vi "Encode JSON Recursive.vi"(4 "error in (no error)":errorcluster, 6 "String In":string, 7 "JSON Tree":variant) -> (0 "error out":errorcluster, 2 "String Out":string)   [LabVIEW 2011, in "i3-json.lvlib"]
uses:
  i3-json.lvlib
  JSON Types/JSON Type.ctl
  Generation Error.ctl
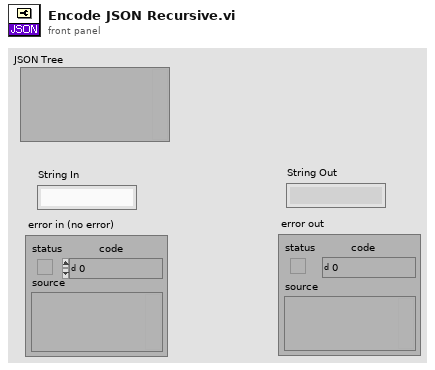
[diagram p1: front panel]
types:
  T1 = typedef "i3-json.lvlib/JSON Type.ctl" = enum8{"JSON Compatible", "JSON Array", "JSON Object", "JSON Null", "Double", "String", "Boolean", "Unknown", "Data JSON string"}
  T2 = typedef "i3-json.lvlib/Generation Error.ctl" = string
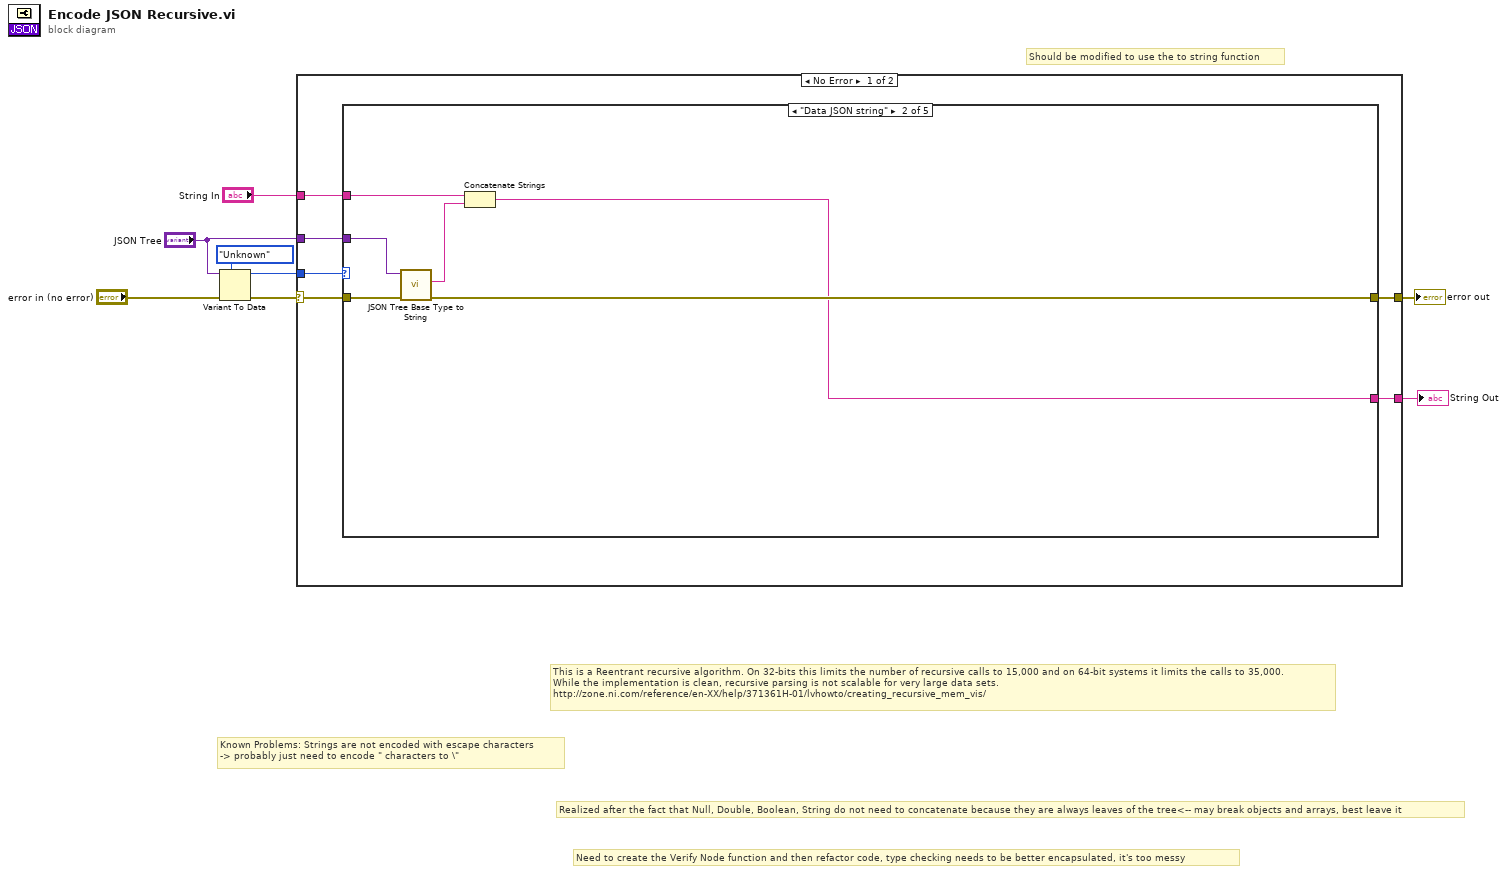
[diagram p0: block diagram]
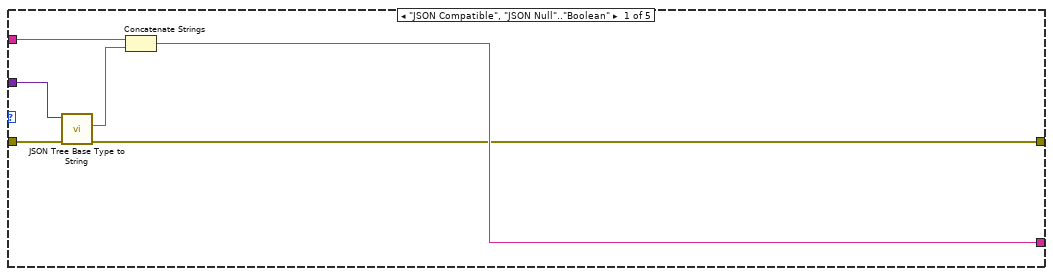
[diagram p2: hidden frame]
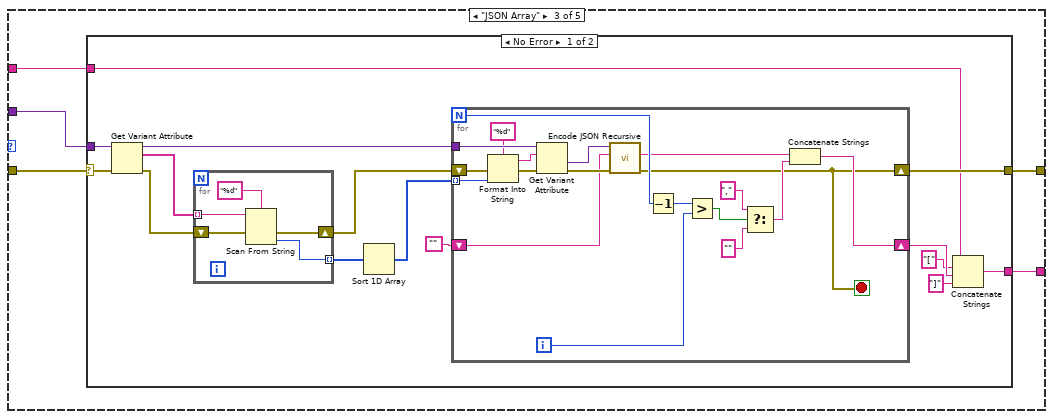
[diagram p3: hidden frame]
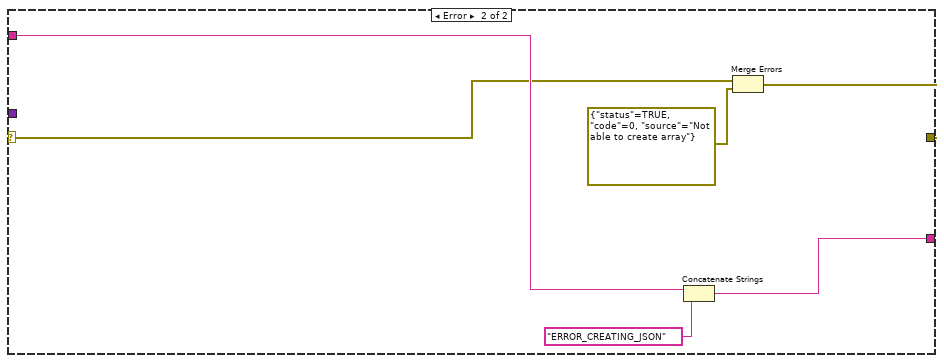
[diagram p4: hidden frame]
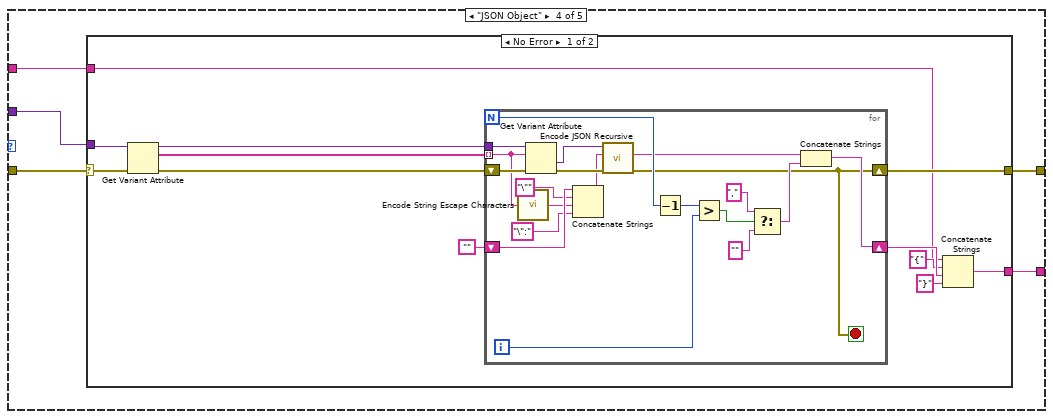
[diagram p5: hidden frame]
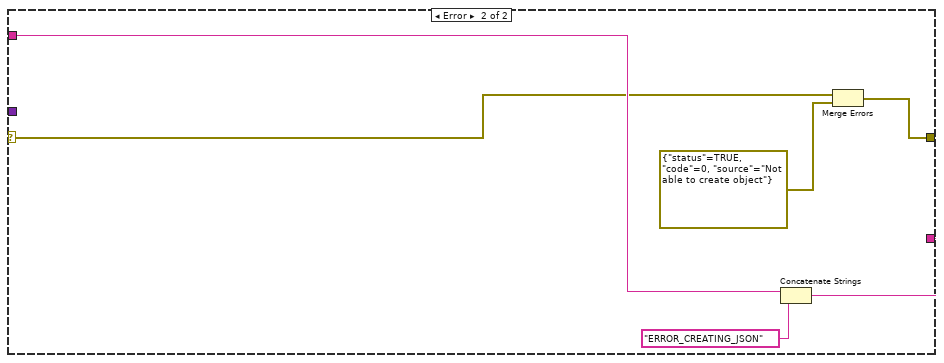
[diagram p6: hidden frame]
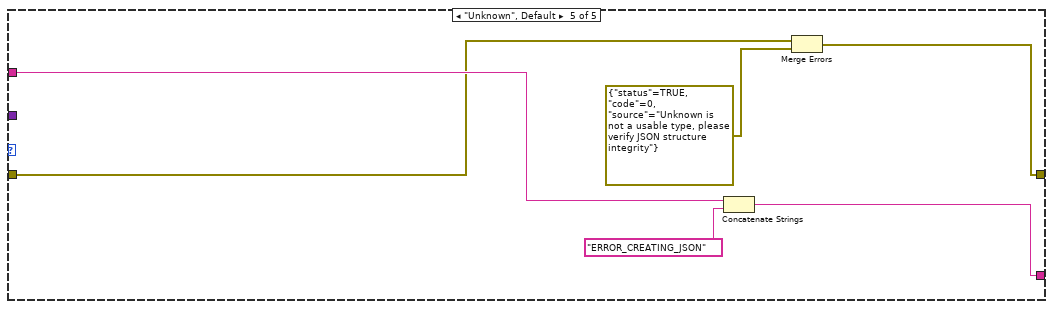
[diagram p7: hidden frame]
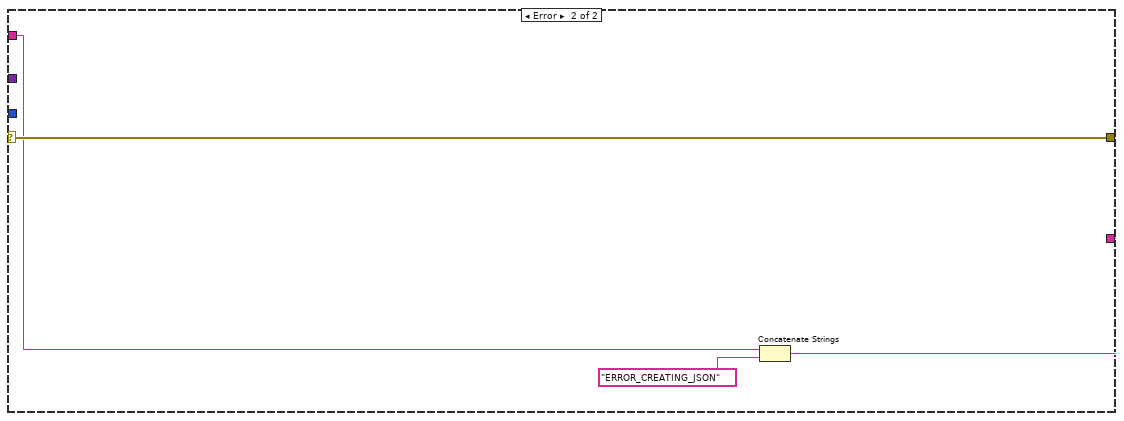
[diagram p8: hidden frame]
diagram:
  # "Should be modified to use the to string function"
  # "Need to create the Verify Node function and then refactor code, type checking needs to be better encapsulated, it's too messy"
  # "Realized after the fact that Null, Double, Boolean, String do not need to concatenate because they are always leaves of the tree<-- may break objects and arrays, best leave it"
  # "Known Problems: Strings are not encoded with escape characters\n-> probably just need to encode \" characters to \\\""
  # "This is a Reentrant recursive algorithm. On 32-bits this limits the number of recursive calls to 15,000 and on 64-bit systems it limits the calls to 35,000.\nWhile the implementation is clean, recursive parsing is not scalable for very large data sets.\nhttp://zone.ni.com/reference/en-XX/help/371361H-01/lvhowto/creating_recursive_mem_vis/"
  n1 = Variant To Data(error in="error in (no error)", type=JSON_Type."Unknown" ("JSON Type"), Variant="JSON Tree") -> (data=w5:T1, error out=w6:errorcluster)
  n2 = case shown="No Error" w6 {
    selector: w6 -> [w12 w129]
    tunnel: w5 -> [w14 _]
    tunnel: "JSON Tree" -> [w13 _]
    tunnel: "String In" -> [w11 w128]
    tunnel: [w10 w127] -> w3
    tunnel: [w9 w129] -> w2
    frame No Error {
      n3 = case shown="\"Data JSON string\"" w14 {
        tunnel: w13 -> [w15 w24 w28 w81 _]
        tunnel: w12 -> [w16 w23 w30 w77 w120]
        tunnel: w11 -> [w20 w25 w29 w80 w124]
        tunnel: [w18 w21 w27 w79 w123] -> w10
        tunnel: [w17 w22 w31 w78 w122] -> w9
        frame "JSON Compatible", "JSON Null".."Boolean" {
          n4 = call "JSON Tree Base Type to String.vi"("error in (no error)"=w16, "JSON Tree Base Type"=w15) -> ("error out"=w17:errorcluster, "JSON Tree Base Type String"=w19:string)  [unwired: 8 in]
          n5 = Concatenate Strings(w20, w19) -> (w18:string)
        }
        frame "Data JSON string" {
          n6 = call "JSON Tree Base Type to String.vi"("error in (no error)"=w23, "JSON Tree Base Type"=w24) -> ("error out"=w22:errorcluster, "JSON Tree Base Type String"=w26:string)  [unwired: 8 in]
          n7 = Concatenate Strings(w25, w26) -> (w21:string)
        }
        frame "JSON Array" {
          n8 = case shown="No Error" w30 {
            selector: w30 -> [w45 w71]
            tunnel: [w42 w76] -> w31
            tunnel: w29 -> [w37 w75]
            tunnel: [w39 w73] -> w27
            tunnel: w28 -> [w46 _]
            frame No Error {
              n9 = Get Variant Attribute(Variant=w46, error in=w45) -> (duplicate Variant=w44:variant, names=w35:string[], error out=w32:errorcluster)  [unwired: 2 in, 1 out]
              n10 = for {
                tunnel: w35 -> [w51] mode=indexing
                shift-right: [w49] -> w33
                shift-left: w32 -> [w50]
                tunnel: [w48] -> w34 mode=indexing
                n11 = Scan From String(format string="%d", input string=w51, error in=w50) -> (error out=w49:errorcluster, output 1=w48:i32)  [unwired: 2 in, 2 out]
              }
              n12 = Sort 1D Array(array=w34) -> (sorted array=w43:i32[])
              n13 = for {
                N -> [w67]
                tunnel: w44 -> [w70]
                tunnel: w43 -> [w54] mode=indexing
                shift-right: [w57] -> w42
                shift-left: w33 -> [w55]
                shift-right: [w59] -> w41
                shift-left: "" -> [w58]
                i -> [w61]
                stop <- w57 stop-if-true
                n14 = Format Into String(format string="%d", error in=w55, w54) -> (resulting string=w52:string, error out=w56:errorcluster)  [unwired: 1 in]
                n15 = Get Variant Attribute(Variant=w70, name=w52, error in=w56) -> (value=w68:variant, error out=w69:errorcluster)  [unwired: 1 in, 2 out]
                n16 = call "Encode JSON Recursive.vi"("error in (no error)"=w69, "String In"=w58, "JSON Tree"=w68) -> ("error out"=w57:errorcluster, "String Out"=w63:string)  [unwired: 3 in]
                n17 = Decrement(x=w67) -> (x-1=w60:i32)
                n18 = Greater?(x=w60, y=w61) -> (0:w66:bool)
                n19 = Select(t=",", s=w66, f="") -> (s? t:f=w62:string)
                n20 = Concatenate Strings(w63, w62) -> (w59:string)
              }
              n21 = Concatenate Strings(w37, "[" ("string"), w41, "]" ("string")) -> (w39:string)
            }
            frame Error {
              n22 = Concatenate Strings(w75, T2 "ERROR_CREATING_JSON" ("Generating Error")) -> (w73:string)
              n23 = Merge Errors(w71, errorcluster {"status"=TRUE, "code"=0, "source"="Not able to create array"} ("error in")) -> (w76:errorcluster)
            }
          }
        }
        frame "JSON Object" {
          n24 = case shown="No Error" w77 {
            selector: w77 -> [w92 w114]
            tunnel: [w89 w119] -> w78
            tunnel: w80 -> [w84 w118]
            tunnel: [w86 w116] -> w79
            tunnel: w81 -> [w93 _]
            frame No Error {
              n25 = Get Variant Attribute(Variant=w93, error in=w92) -> (duplicate Variant=w91:variant, names=w83:string[], error out=w90:errorcluster)  [unwired: 2 in, 1 out]
              n26 = for {
                N -> [w109]
                tunnel: w91 -> [w113]
                shift-right: [w96] -> w89
                shift-left: w90 -> [w112]
                shift-right: [w101] -> w88
                shift-left: "" -> [w100]
                tunnel: w83 -> [w94] mode=indexing
                i -> [w103]
                stop <- w96 stop-if-true
                n27 = call "Encode String Escape Characters.vi"("unescaped string in"=w94) -> ("escaped string out"=w95:string)
                n28 = Get Variant Attribute(Variant=w113, name=w94, error in=w112) -> (value=w110:variant, error out=w111:errorcluster)  [unwired: 1 in, 2 out]
                n29 = Concatenate Strings(w100, "\"" ("string"), w95, "\":" ("string")) -> (w97:string)
                n30 = call "Encode JSON Recursive.vi"("error in (no error)"=w111, "String In"=w97, "JSON Tree"=w110) -> ("error out"=w96:errorcluster, "String Out"=w105:string)  [unwired: 3 in]
                n31 = Decrement(x=w109) -> (x-1=w102:i32)
                n32 = Greater?(x=w102, y=w103) -> (0:w108:bool)
                n33 = Select(t=",", s=w108, f="") -> (s? t:f=w104:string)
                n34 = Concatenate Strings(w105, w104) -> (w101:string)
              }
              n35 = Concatenate Strings(w84, "{" ("string"), w88, "}" ("string")) -> (w86:string)
            }
            frame Error {
              n36 = Concatenate Strings(w118, T2 "ERROR_CREATING_JSON" ("Generating Error")) -> (w116:string)
              n37 = Merge Errors(w114, errorcluster {"status"=TRUE, "code"=0, "source"="Not able to create object"} ("error in")) -> (w119:errorcluster)
            }
          }
        }
        frame "Unknown", Default {
          n38 = Concatenate Strings(w124, T2 "ERROR_CREATING_JSON" ("Generating Error")) -> (w123:string)
          n39 = Merge Errors(w120, errorcluster {"status"=TRUE, "code"=0, "source"="Unknown is not a usable type, please verify JSON structure integrity"} ("error in")) -> (w122:errorcluster)
        }
      }
    }
    frame Error {
      n40 = Concatenate Strings(w128, T2 "ERROR_CREATING_JSON" ("string")) -> (w127:string)
    }
  }
  "String Out" <- w3
  "error out" <- w2
